vi "2D Gaussian - Function -init.vi"(3 "output control":T1, 4 "data":T2, 5 "X":dbl[](array[numeric]), 6 "a":dbl[](array[numeric])) -> (0 "error out":errorcluster, 1 "f'(X,a)":dbl[][](array[numeric]), 2 "f(X,a)":dbl[](array[numeric]))   [LabVIEW 2016]
doc: "This template is the starting point for creating a model function to be passed to the Nonlinear Curve Fit.vi."
uses:
  <vilib>/gmath/NumericalOptimization/objective function data.ctl
  <vilib>/gmath/NumericalOptimization/LM_output select.ctl
  <vilib>/gmath/NI_Gmath.lvlib
panel:
  # "Amp\nXo\nYo\nWx\nWy\nOffset"
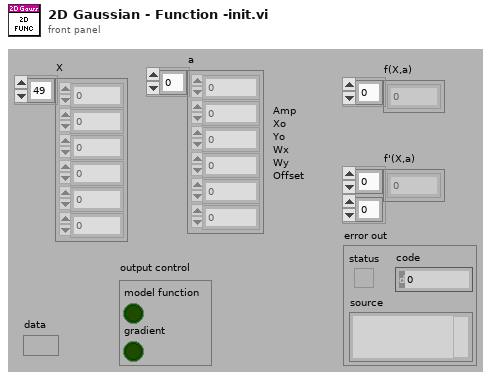
[diagram p1: front panel]
types:
  T1 = typedef "NI_Gmath.lvlib/LM_output select.ctl" = cluster{"model function":bool, "gradient":bool}
  T2 = typedef "NI_Gmath.lvlib/objective function data.ctl" = variant
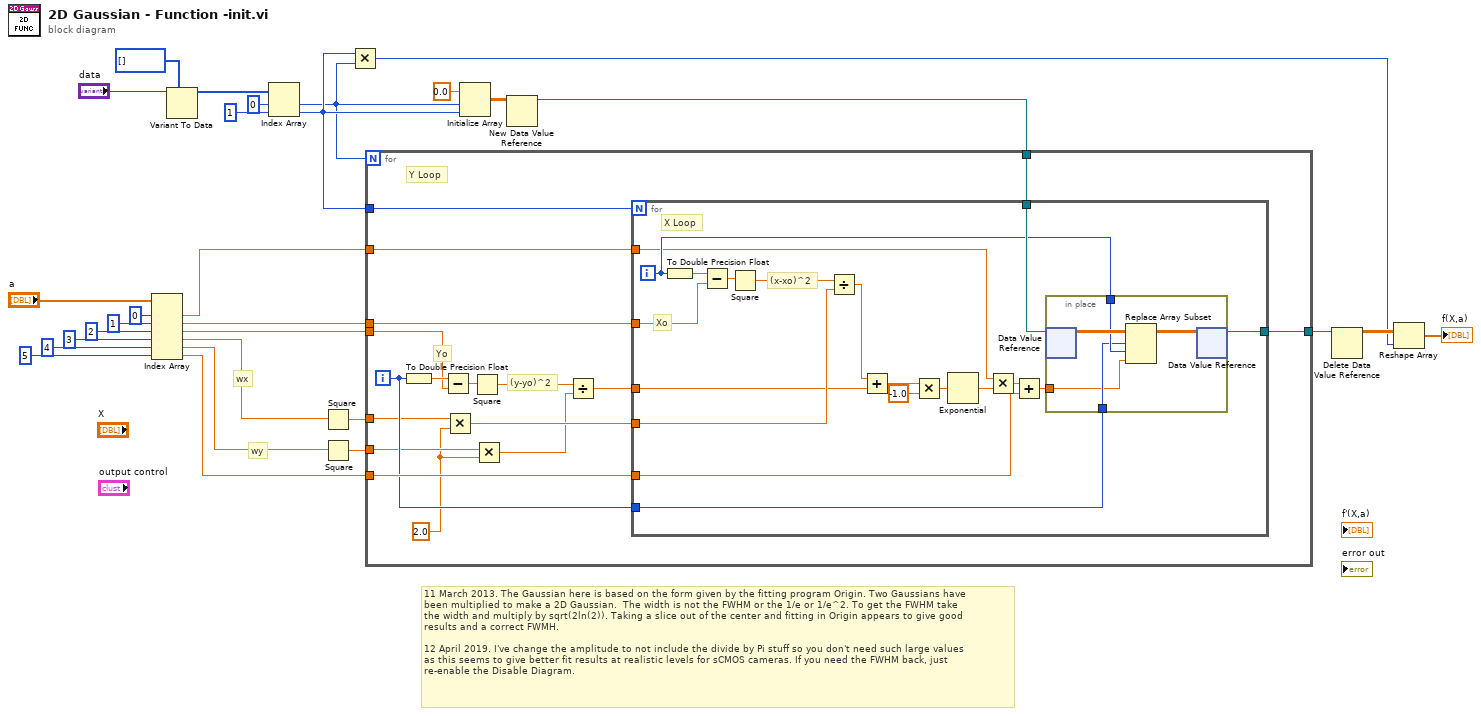
[diagram p0: block diagram]
diagram:
  # "11 March 2013. The Gaussian here is based on the form given by the fitting program Origin. Two Gaussians have\nbeen multiplied to make a 2D Gaussian.  The width is not the FWHM or the 1/e or 1/e^2. To get the FWHM take\nthe width and multiply by sqrt(2ln(2)). Taking a slice out of the center and fitting in Origin appears to give good\nresults and a correct FWMH.\n\n12 April 2019. I've change the amplitude to not include the divide by Pi stuff so you don't need such large values\nas this seems to give better fit results at realistic levels for sCMOS cameras. If you need the FWHM back, just\nre-enable the Disable Diagram."
  # "wy"
  # "wx"
  n1 = Index Array(array="a", index #1=0 ("index"), index #2=1 ("index"), index #3=2 ("index"), index #4=3 ("index"), index #5=4 ("index"), index #6=5 ("index")) -> (element #1=w1:dbl, element #2=w28:dbl, element #3=w27:dbl, element #4=w18:dbl, element #5=w17:dbl, element #6=w26:dbl)
  n2 = Variant To Data(type=i32[] [], Variant="data") -> (data=w13:i32[])  [unwired: 1 in, 1 out]
  n3 = Index Array(array=w13, index #1=0 ("index"), index #2=1 ("index")) -> (element #1=w8:i32, element #2=w9:i32)
  n4 = Square(x=w18) -> (x^2=w20:dbl)
  n5 = Square(x=w17) -> (x^2=w19:dbl)
  n6 = Multiply(x=w9, y=w8) -> (x*y=w10:i32)
  n7 = Initialize Array(0.0 ("element"), w8, w9) -> (w24:dbl[][])
  n8 = New Data Value Reference(data value=w24) -> (data value reference=w23:refnum<data-value>)  [unwired: 1 in, 1 out]
  n9 = for {
    N: w8 -> [_]
    tunnel: w28 -> [w46]
    tunnel: w27 -> [w43]
    tunnel: w26 -> [w45]
    tunnel: w23 -> [w41]
    tunnel: [w39] -> w22
    tunnel: w20 -> [w34]
    tunnel: w19 -> [w32]
    tunnel: w1 -> [w36]
    tunnel: w9 -> [w35]
    i -> [w40]
    w30 = 2.0 ("y")
    # "(y-yo)^2"
    # "Yo"
    # "Y Loop"
    n10 = To Double Precision Float(number=w40) -> (double precision float=w44:dbl)
    n11 = Subtract(x=w44, y=w43) -> (x-y=w42:dbl)
    n12 = Multiply(x=w34, y=w30) -> (x*y=w33:dbl)
    n13 = Square(x=w42) -> (x^2=w38:dbl)
    n14 = Multiply(x=w32, y=w30) -> (x*y=w31:dbl)
    n15 = Divide(x=w38, y=w31) -> (x/y=w37:dbl)
    n16 = for {
      N: w35 -> [_]
      tunnel: w46 -> [w64]
      tunnel: w45 -> [w62]
      tunnel: w41 -> [w61]
      tunnel: w40 -> [w59]
      tunnel: [w57] -> w39
      tunnel: w33 -> [w55]
      tunnel: w37 -> [w54]
      tunnel: w36 -> [w47]
      i -> [w60]
      # "Xo"
      # "(x-xo)^2"
      # "X Loop"
      n17 = To Double Precision Float(number=w60) -> (double precision float=w65:dbl)
      n18 = Subtract(x=w65, y=w64) -> (x-y=w63:dbl)
      n19 = Square(x=w63) -> (x^2=w56:dbl)
      n20 = Divide(x=w56, y=w55) -> (x/y=w53:dbl)
      n21 = Add(x=w53, y=w54) -> (x+y=w52:dbl)
      n22 = Multiply(x=w52, y=-1.0) -> (x*y=w50:dbl)
      n23 = Exponential(1:w50) -> (0:w49:dbl)
      n24 = Multiply(x=w47, y=w49) -> (x*y=w48:dbl)
      n25 = Add(x=w48, y=w62) -> (x+y=w58:dbl)
      n26 = in-place {
        in-place-border: w60 -> [w68]
        in-place-border: w59 -> [w67]
        in-place-border: w58 -> [w66]
        n27 = in-place-dvr #1(w61) -> (w70:dbl[][])  [unwired: 1 out]
        n28 = Replace Array Subset(array=w70, new element=w66, index (row)=w67, index (col)=w68) -> (w69:dbl[][])
        n29 = in-place-dvr #1(w69) -> (w57:refnum<data-value>)  [unwired: 1 out]
      }
    }
  }
  n30 = Delete Data Value Reference(data value reference=w22) -> (data value=w16:dbl[][])  [unwired: 1 in, 1 out]
  n31 = Reshape Array(w16, w10) -> (→"f(X,a)":dbl[])
